vi "Default Instrument Setup.vi"(8 "error in (no error)":errorcluster, 11 "VISA resource name":refnum<visa-resource-name>) -> (0 "error out":errorcluster, 3 "VISA resource name out":refnum<visa-resource-name>)   [LabVIEW 2024, in "Keithley 2200 Series.lvlib"]
doc: "This Utility VI sends a default command string to the instrument whenever a new VISA session is opened, or the instrument is reset. Use this VI as a subVI for the Initialize and Reset VIs. Altering this VI could cause these two VIs to operate incorrectly"
uses:
  Keithley 2200 Series.lvlib
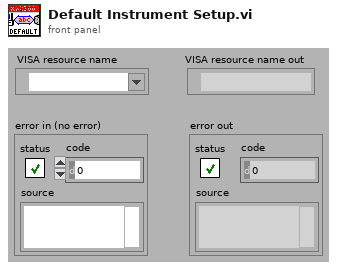
[diagram p1: front panel]
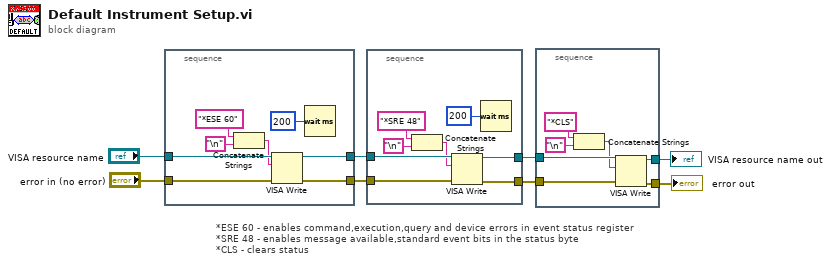
[diagram p0: block diagram]
diagram:
  # "*ESE 60 - enables command,execution,query and device errors in event status register\n*SRE 48 - enables message available,standard event bits in the status byte\n*CLS - clears status"
  n1 = stacked-sequence {
    tunnel: "VISA resource name" -> [w16]
    tunnel: "error in (no error)" -> [w15]
    tunnel: [w13] -> w6
    tunnel: [w12] -> w5
    frame #0 {
      n2 = Concatenate Strings("*ESE 60" ("write buffer"), "\n") -> (w9:string)
      n3 = VISA Write(VISA resource name=w16, write buffer=w9, error in (no error)=w15) -> (VISA resource name out=w13:refnum<visa-resource-name>, error out=w12:errorcluster)  [unwired: 1 out]
      n4 = Wait (ms)(milliseconds to wait=u32 200) -> ()  [unwired: 1 out]
    }
  }
  n5 = stacked-sequence {
    tunnel: w6 -> [w23]
    tunnel: w5 -> [w22]
    tunnel: [w21] -> w4
    tunnel: [w20] -> w3
    frame #0 {
      n6 = Concatenate Strings("*SRE 48" ("write buffer"), "\n") -> (w17:string)
      n7 = VISA Write(VISA resource name=w23, write buffer=w17, error in (no error)=w22) -> (VISA resource name out=w21:refnum<visa-resource-name>, error out=w20:errorcluster)  [unwired: 1 out]
      n8 = Wait (ms)(milliseconds to wait=u32 200) -> ()  [unwired: 1 out]
    }
  }
  n9 = stacked-sequence {
    tunnel: w4 -> [w31]
    tunnel: w3 -> [w30]
    tunnel: [w29] -> w2
    tunnel: [w28] -> w1
    frame #0 {
      n10 = Concatenate Strings("*CLS" ("write buffer"), "\n") -> (w25:string)
      n11 = VISA Write(VISA resource name=w31, write buffer=w25, error in (no error)=w30) -> (VISA resource name out=w29:refnum<visa-resource-name>, error out=w28:errorcluster)  [unwired: 1 out]
    }
  }
  "VISA resource name out" <- w2
  "error out" <- w1
